vi "Temperature Monitor.vi"() -> ()   [LabVIEW 2018]
doc: "이 VI는 LabVIEW Core I 교육 과정의 연습문제에 대한 해답입니다.\n\n이 VI는 While 루프와 시프트 레지스터를 사용하여 데이터의 평균을 구합니다. 하드웨어는 필요하지 않습니다."
panel:
  in  "정지 버튼":bool
  out "온도 히스토리":cluster{dbl, "온도 값":dbl}(graph)
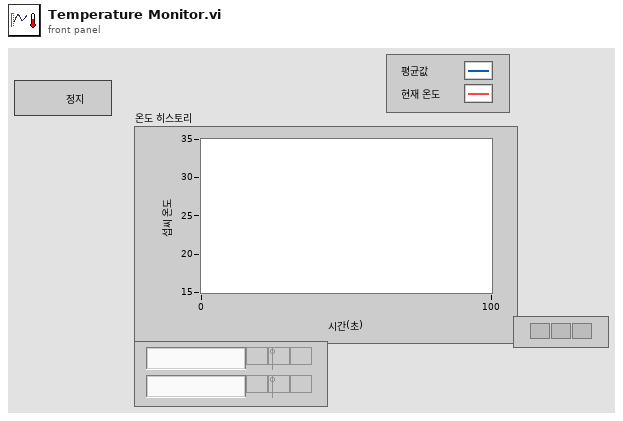
[diagram p1: front panel]
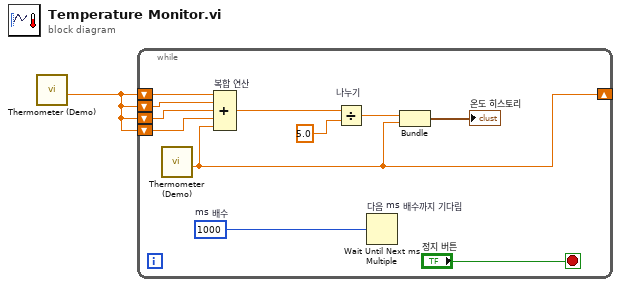
[diagram p0: block diagram]
diagram:
  n1 = call "Thermometer (Demo).vi"() -> ("온도 값"=w1:dbl)  [unwired: 11 in]
  n2 = while {
    shift-right: [w3] -> _
    shift-left: w1 -> [w10]
    shift-left: w1 -> [w9]
    shift-left: w1 -> [w8]
    shift-left: w1 -> [w7]
    stop <- "정지 버튼" stop-if-true
    w12 = u32 1000  # ms 배수
    n3 = call "Thermometer (Demo).vi"() -> ("온도 값"=w3:dbl)  [unwired: 11 in]
    n4 = Compound Arithmetic op=ADD "복합 연산"(w10, w9, w8, w7, w3) -> (w6:dbl)
    n5 = Divide "나누기"(x=w6, y=5.0) -> (x/y=w4:dbl)
    n6 = Wait Until Next ms Multiple "다음 ms 배수까지 기다림"(millisecond multiple=w12) -> ()  [unwired: 1 out]
    n7 = Bundle(w4, "온도 값"=w3) -> (→"온도 히스토리":cluster{dbl, "온도 값":dbl})  [unwired: 1 in]
  }
